vi "ExamineImageCalibration.vi"(0 "Calibration Image":path=path "E:/XYZstage+Camera_CollectedImages/12-12-2016/Calibration_moduleOnStave_0,2p2,0.png", 11 "error in (no error)":errorcluster) -> (1 "Error Map":sgl[][](array[numeric]) format="%.2f", 3 "User ROI Descriptor":T1 {"Contours"."Type" items=["No Selection", "Point", "Line", "Rectangle", "Oval", "Polygon", "Freehand Region", "Annulus", "Unused2", "Unused3", "Broken Line", "Freehand Line", "Rotated Rectangle"]}, 4 "Calibration Image out":T8(plugin-control), 6 "Calibration Axis Info":T2={"Origin Pixel"={"X"=0.0, "Y"=0.0}, "Angle Relative to Horizontal (deg)"=0.0, "X Axis Pixel"={"X"=0.0, "Y"=0.0}, "Axis Reference"=1} {"X Axis Pixel"."Y" format="%.2f"; "X Axis Pixel"."X" format="%.2f"; "Axis Reference" items=["Direct", "Indirect"]; "Angle Relative to Horizontal (deg)" format="%.2f"; "Origin Pixel"."Y" format="%.2f"; "Origin Pixel"."X" format="%.2f"}, 8 "Error Statistics":T7, 10 "Calibration Learn Setup":T5={"Method"=4, "Distortion"=-1, "Corrected Image Scaling"=0, "Corrected Image Learn ROI"=0, "Learn Correction Table?"=FALSE} {"Distortion" items=["None"=-1, "Polynomial"=0, "Division"=1]; "Corrected Image Learn ROI" items=["Full Image ", "Calibration ROI", "ROI", "Calibration AND ROI", "Calibration OR ROI"]; "Corrected Image Scaling" items=["Scale to Preserve Area", "Scale to Fit"]; "Method" items=["Perspective", "Microplane", "Simple", "Corrected", "None"]}, 12 "Grid Descriptor":T3={"X Step"=1.0, "Y Step"=1.0, "Unit"=enum."Undefined"} {"Y Step" format="%.2f"; "X Step" format="%.2f"}, 14 "Calibration ROI Descriptor":T1 {"Contours"."Type" items=["No Selection", "Point", "Line", "Rectangle", "Oval", "Polygon", "Freehand Region", "Annulus", "Unused2", "Unused3", "Broken Line", "Freehand Line", "Rotated Rectangle"]}, 15 "error out":errorcluster)   [LabVIEW 2016]
uses:
  <vilib>/vision/Calibration.llb/Error Statistics.ctl
  <vilib>/vision/Calibration.llb/Correction Learn Setup.ctl
  <vilib>/vision/Calibration.llb/Distortion Model Types.ctl
  <vilib>/vision/NI_Vision_Development_Module.lvlib
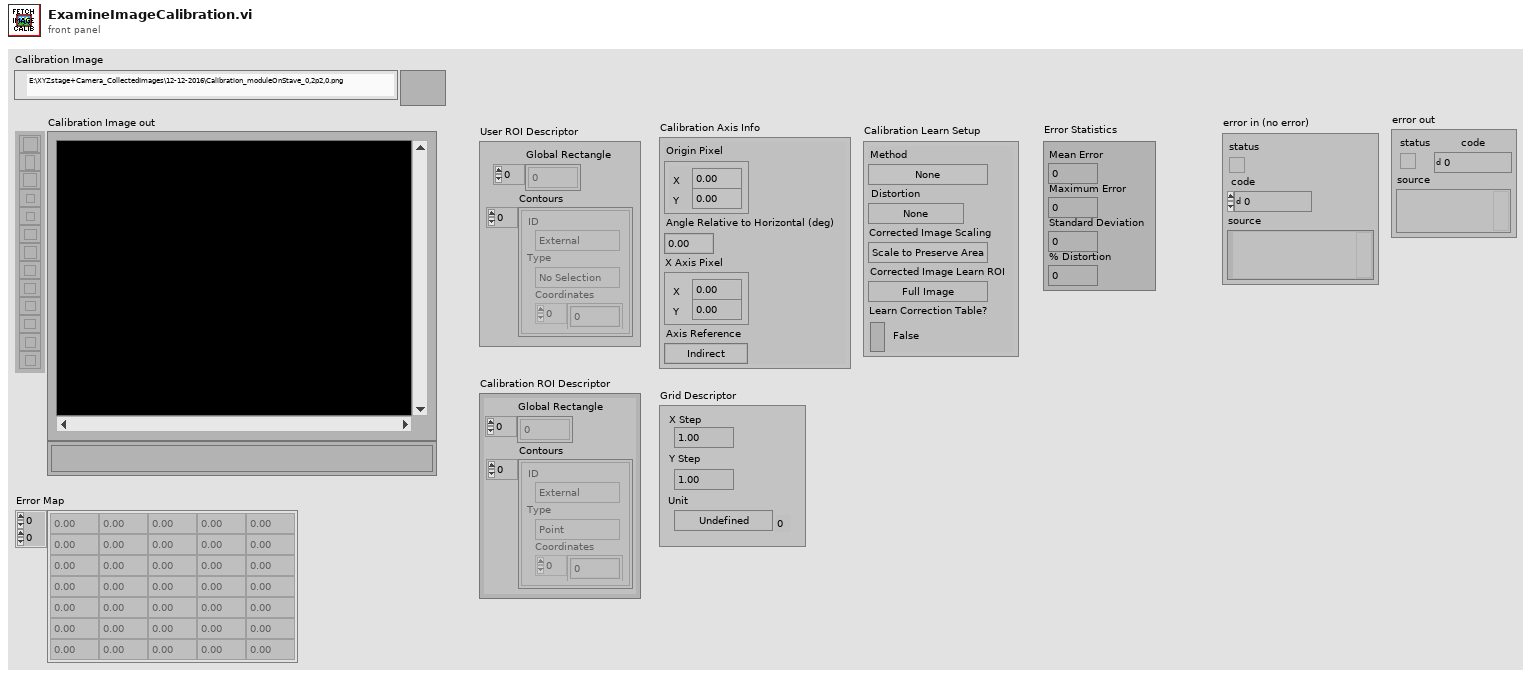
[diagram p1: front panel]
types:
  T1 = typedef "ROI Descriptor" = cluster{"Global Rectangle":i32[], "Contours":cluster{"ID":enum32{"External", "Internal"}, "Type":u32, "Coordinates":i32[]}[]}
  T2 = cluster{"Origin Pixel":cluster{"X":sgl, "Y":sgl}, "Angle Relative to Horizontal (deg)":sgl, "X Axis Pixel":cluster{"X":sgl, "Y":sgl}, "Axis Reference":u32}
  T3 = typedef "Simple Grid Descriptor" = cluster{"X Step":sgl, "Y Step":sgl, "Unit":T4}
  T4 = typedef "Image Unit" = enum32{"Undefined", "Angström", "Micrometer", "Millimeter", "Centimeter", "Meter", "Kilometer", "Microinch", "Inch", "Feet", "Nautical miles", "Standard miles", "Steps"}
  T5 = typedef "Correction Learn Setup.ctl" = cluster{"Method":u32, "Distortion":T6, "Corrected Image Scaling":u32, "Corrected Image Learn ROI":u32, "Learn Correction Table?":bool}
  T6 = typedef "Distortion Model Types.ctl" = i32
  T7 = typedef "Error Statistics.ctl" = cluster{"Mean Error":dbl, "Maximum Error":dbl, "Standard Deviation":dbl, "% Distortion":dbl}
  T8 = typedef "IMAQ Image.ctl" = refnum<image>
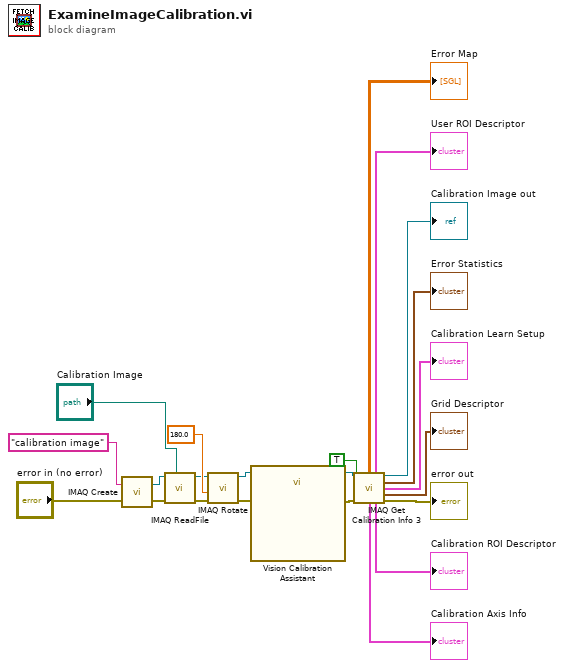
[diagram p0: block diagram]
diagram:
  n1 = call "IMAQ Create"("Image Name"="calibration image", "error in (no error)"="error in (no error)") -> ("New Image"=w5:T8, "error out"=w4:errorcluster)  [unwired: 3 in]
  n2 = call "IMAQ ReadFile"("File Path"="Calibration Image", "error in (no error)"=w4, "Image"=w5) -> ("error out"=w9:errorcluster, "Image Out"=w10:T8)  [unwired: 4 in, 3 out]
  n3 = call "IMAQ Rotate"("error in (no error)"=w9, "Angle (degrees)"=sgl 180.0, "Image Src"=w10) -> ("error out"=w13:errorcluster, "Image Dst Out"=w12:T8)  [unwired: 7 in]
  n4 = call "Vision Calibration Assistant"("Image In"=w12, "error in"=w13) -> ("Image Out"=w14:T8, "error out"=w3:errorcluster)  [unwired: 24 in]
  n5 = call "IMAQ Get Calibration Info 3"("Calibration Template Image"=w14, "Return Error Information (False)"=TRUE, "error in (no error)"=w3) -> ("Error Map"=→"Error Map":sgl[][], "User ROI Descriptor"=→"User ROI Descriptor":T1, "Calibration Template Image (duplicate)"=→"Calibration Image out":T8, "Error Statistics"=→"Error Statistics":T7, "Calibration Learn Setup"=→"Calibration Learn Setup":T5, "Grid Descriptor"=→"Grid Descriptor":T3, "Calibration Axis Info"=→"Calibration Axis Info":T2, "Calibration ROI Descriptor"=→"Calibration ROI Descriptor":T1, "error out"=→"error out":errorcluster)  [unwired: 4 in]
